vi "RSZVB Get IF Gain.vi"(8 "error in (no error)":errorcluster {"code" format="%.0x"}, 9 "Port (1)":i32=1, 10 "Channel (1)":i32=1, 11 "VISA session":refnum<visa-resource-name>) -> (0 "error out":errorcluster {"code" format="%.0x"}, 2 "IF Gain":i32, 3 "dup VISA session":refnum<visa-resource-name>)   [LabVIEW 2011]
doc: "This VI returns the IF gain in the measurement channel b. \n\nRemote-control command(s):\n[SENSe<Ch>:]POWer:IFGain<Pt>:MEASure?"
uses:
  _utility/RSZVB Global Data.vi
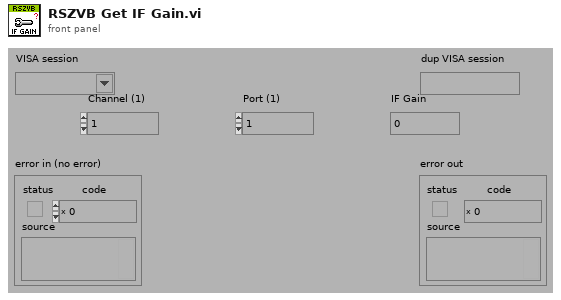
[diagram p1: front panel]
types:
  T1 = cluster{"Error Checking (T: On)":bool, "Installed Options":string[], "Data Valid?":bool, "Ports":i32, "Model":string[], "Option Checking (T: On)":bool}[]
  T2 = cluster{"Error Checking (T: On)":bool, "Installed Options":string[], "Data Valid?":bool, "Ports":i32, "Model":string[], "Option Checking (T: On)":bool}
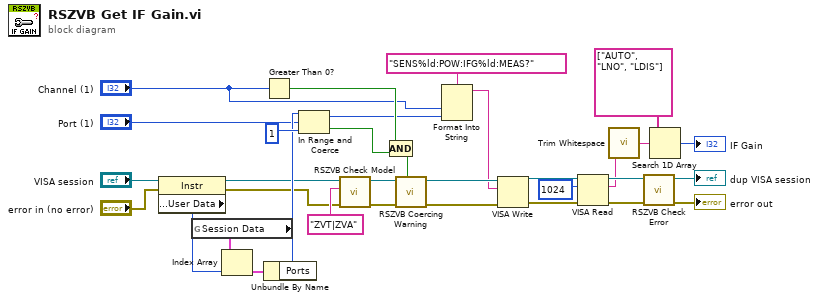
[diagram p0: block diagram]
diagram:
  n1 = property class="Instr"(reference="VISA session", error in="error in (no error)") -> (reference out=w1:refnum<visa-resource-name>, error out=w4:errorcluster, "General Settings:User Data"=w24:u32)
  n2 = global read "RSZVB Global Data.vi" "Session Data"() -> (w25:T1)
  n3 = Index Array(array=w25, index=w24) -> (element=w26:T2)
  n4 = Greater Than 0?(x="Channel (1)") -> (x > 0?=w27:bool)
  n5 = Unbundle By Name(w26) -> ("Ports"=w23:i32)
  n6 = In Range and Coerce(upper limit=w23, x="Port (1)", lower limit=1) -> (coerced(x)=w21:i32, In Range?=w22:bool)
  n7 = call "RSZVB Check Model.vi"("error in (no error)"=w4, "Model"="ZVT|ZVA" ("Options"), "VISA session"=w1) -> ("error out"=w3:errorcluster, "dup VISA session"=w2:refnum<visa-resource-name>)  [unwired: 7 in]
  n8 = Compound Arithmetic op=AND(w27, w22) -> (w29:bool)
  n9 = call "RSZVB Coercing Warning.vi"("In Range?"=w29, "error in (no error)"=w3, "VISA session"=w2) -> ("error out"=w30:errorcluster, "dup VISA session"=w31:refnum<visa-resource-name>)  [unwired: 7 in]
  n10 = Format Into String(format string="SENS%ld:POW:IFG%ld:MEAS?", "Channel (1)", w21) -> (resulting string=w28:string)  [unwired: 2 in, 1 out]
  n11 = VISA Write(VISA resource name=w31, write buffer=w28, error in (no error)=w30) -> (VISA resource name out=w12:refnum<visa-resource-name>, error out=w13:errorcluster)  [unwired: 1 out]
  n12 = VISA Read(VISA resource name=w12, byte count=u32 1024 ("byte count (0)"), error in (no error)=w13) -> (VISA resource name out=w15:refnum<visa-resource-name>, read buffer=w11:string, error out=w14:errorcluster)  [unwired: 1 out]
  n13 = call <vilib>:"Trim Whitespace.vi"("string"=w11) -> ("trimmed string"=w8:string)  [unwired: 1 in]
  n14 = call "RSZVB Check Error.vi"("error in (no error)"=w14, "VISA session"=w15) -> ("error out"=→"error out":errorcluster, "dup VISA session"=→"dup VISA session":refnum<visa-resource-name>)  [unwired: 8 in]
  n15 = Search 1D Array(1D array=string[] ["AUTO", "LNO", "LDIS"] ("array 2"), element=w8) -> (index of element=→"IF Gain":i32)  [unwired: 1 in]
